vi "TDMS Playback Functional.vi"(1 "Scale Factor Linear":dbl=1.1934598400763813e-07, 4 "IQ Swap Enabled":bool=TRUE, 5 "IQ Rate (S/s)":dbl=25000000.0 format="%#_3p", 6 "pre filter gain":dbl, 7 "channel name (iq/qi)":string="qi", 8 "error in":errorcluster={"status"=FALSE, "code"=373504, "source"="niRFSG Close.vi<ERR>DSP overflow detected. The output waveform was clipped. Reduce the Arb Pre-filter Gain to eliminate overflow."}, 9 "Output Power (dBm)":dbl=10.0 format="%#_3p", 10 "Carrier (Hz)":dbl=3550000000.0 format="%#_3p", 11 "Path":path) -> (0 "error out":errorcluster={"status"=FALSE, "code"=373504, "source"="niRFSG Close.vi<ERR>DSP overflow detected. The output waveform was clipped. Reduce the Arb Pre-filter Gain to eliminate overflow."}, 2 "Playback Progress":i32(slide)=383 scale=-1.0..536.0)   [LabVIEW 2017]
uses:
  <instrlib>/niRFSG/niRFSG.llb/niRFSG Write Arb Waveform (Complex DBL).vi
  MainVI/GlobalVariableS.vi
  <vilib>/FPGAPlugInAG/Dynamic/niLvFpga_Close_Dynamic.vi
  <vilib>/rvi/interface/nirviCloseFPGA/nirviCloseFPGA.xnode
panel:
  out "result string 2":string
  out "20 log (scale Factor_Linear)":dbl=-138.46384380841334
  in  "RF:LO Out Enabled":bool
  in  "RF:External Gain (dB)":dbl
  in  "RF:Peak Power Adjustment (dB)":dbl
  out "samples":u32=769639589
  out "number of pending reads 1":u32=8
  out "empty elements":u32=134217728
  out "dma fullness":u32=48764
  out "number of pending reads 2":u32=1
  out "# of elements in host buffer avail for writing":u32=65536
  out "peak fullness":u32
  out "fullness":u32=65536
  out "Completion Loop":i32=3891
  out "fpga peak":u32(slide)=272 scale=-1.0..65536.0
  in  "Monitor Buffer Fullness":bool=TRUE
  out "file peak":u32(slide)=2 scale=0.0..8.0
  out "host peak":u32(slide)=1024 scale=-1.0..134217728.0
  out "File Read Buffer Fullness":u32(slide)=1 scale=0.0..8.0
  out "DMA Host Buffer Emptiness":u32(slide) scale=-1.0..134217728.0
  out "DMA FPGA Buffer Emptiness":u32(slide)=424 scale=-1.0..65536.0
  out "Underflow Detected":bool
  in  "stop button":bool
  in  "Read Block Size (MB)":u32=32 caption="Chunk Size (S)" format="%.0f MB"
  in  "chunks":u32=16 caption="DMA Host Buffer Depth (Blocks)" format="%.0p"
  in  "VST Resource":string="VST"
  # "RF Playback Configuration"
  # "VST Internal FPGA Status"
  # "File"
  # "Current"
  # "Peak"
  # "Current"
  # "Peak"
  # "RF"
  # "Current"
  # "Peak"
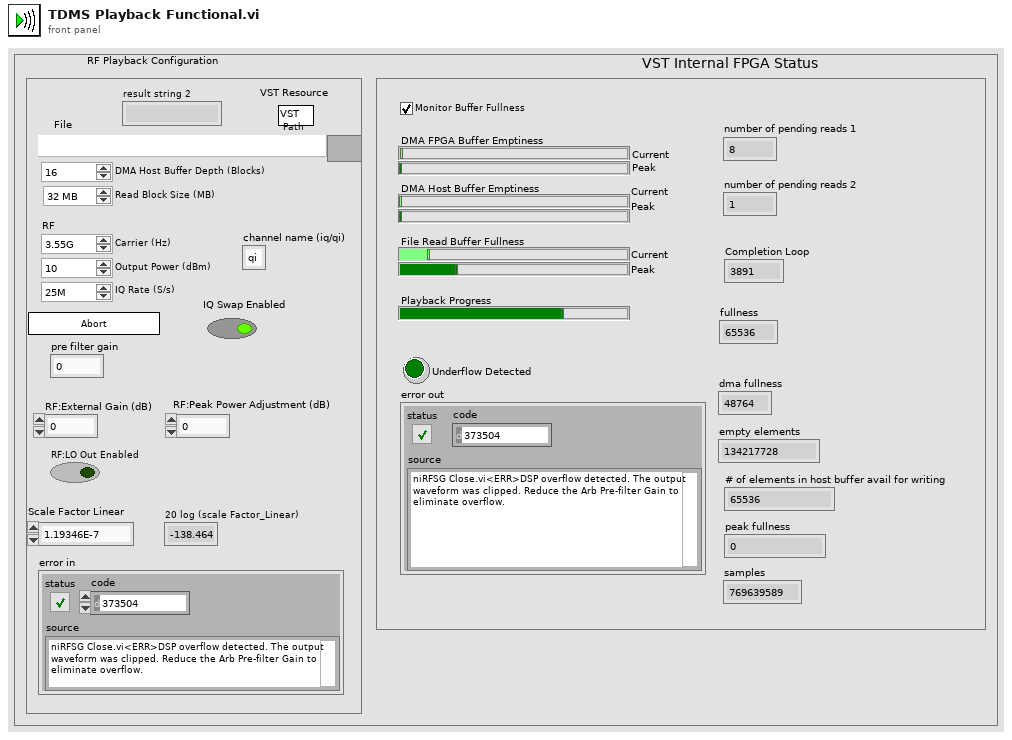
[diagram p1: front panel]
types:
  T1 = enum16{"open", "open or create", "create or replace", "create", "open (read-only)"}
  T2 = cluster{"underflow":bool, "underflows":u32, "samples":u32}
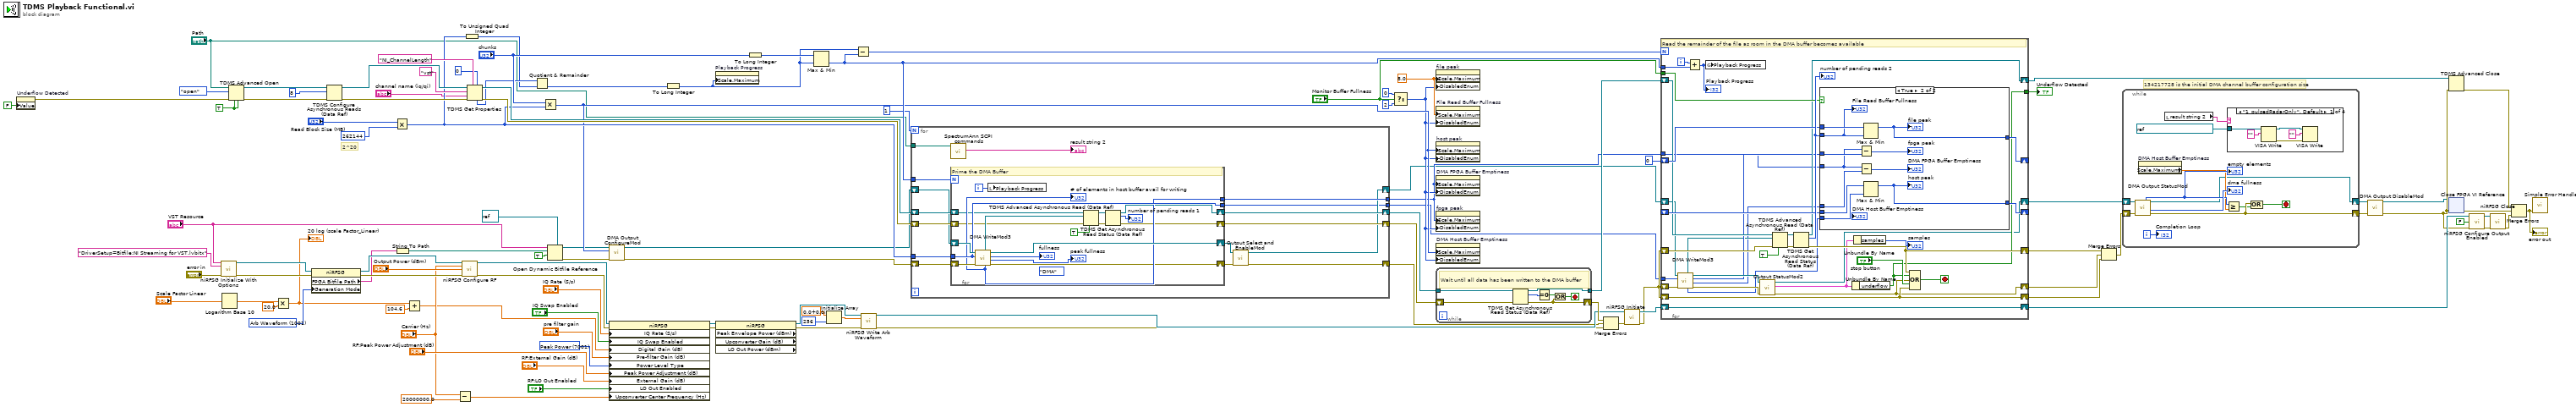
[diagram p0: block diagram]
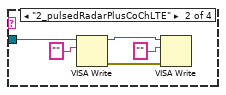
[diagram p3: hidden frame]
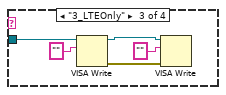
[diagram p4: hidden frame]
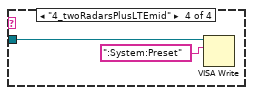
[diagram p5: hidden frame]
diagram:
  w24 = 7001 items=["Average Power"=7000, "Peak Power"=7001] ("RF:Power Level Type")
  w48 = 8.0 ("Scale.Range:Maximum")
  w14 = TRUE ("disable buffering? (T)")
  w102 = 1001 items=["CW"=1000, "Arb Waveform"=1001, "Script"=1002] ("Arb:Generation Mode")
  # "134217728 is the initial DMA channel buffer configuration size"
  # "2^20"
  n1 = property on="Underflow Detected" class="Bool (strict)"("Value"=FALSE ("Underflow Detected")) -> (error out=w46:errorcluster)  [unwired: 2 in, 1 out]
  n2 = call <instrlib>:"niRFSG Initialize With Options.vi"("resource name"="VST Resource", "option string"="DriverSetup=Bitfile:NI Streaming for VST.lvbitx", "error in"="error in") -> ("instrument handle"=w107:refnum<k15>, "error out"=w108:errorcluster)  [unwired: 11 in]
  n3 = Logarithm Base 10(1:"Scale Factor Linear") -> (0:w9:dbl)
  n4 = TDMS Advanced Open(4:w14, 6:w14, 8:w46, 10:T1."open" ("operation (0:open)"), 11:"Path") -> (0:w98:errorcluster, 3:w97:refnum<k34>)  [unwired: 1 out]
  n5 = Multiply(x=w9, y=20.0) -> (x*y=w8:dbl)
  "20 log (scale Factor_Linear)" <- w8
  n6 = property class="niRFSG"(reference=w107, error in=w108, "Generation Mode"=w102) -> (reference out=w105:refnum<k15>, error out=w106:errorcluster, "FPGA Bitfile Path"=w104:string)
  n7 = TDMS Configure Asynchronous Reads (Data Ref)(8:w98, 10:u32 8 ("max asynchronous reads (4)"), 11:w97) -> (0:w87:errorcluster, 3:w88:refnum<k34>)  [unwired: 2 in]
  n8 = Multiply(x="Read Block Size (MB)", y=u32 262144) -> (x*y=w56:u32)
  n9 = String To Path(string=w104) -> (path=w36:path)
  n10 = Add(x=w8, y=104.6) -> (x+y=w4:dbl)
  n11 = Subtract(x="Carrier (Hz)", y=20000000.0) -> (x-y=w10:dbl)
  n12 = call <instrlib>:"niRFSG Configure RF.vi"("instrument handle"=w105, "frequency (Hz)"="Carrier (Hz)", "power level (dBm)"="Output Power (dBm)", "error in"=w106) -> ("instrument handle out"=w23:refnum<k15>, "error out"=w22:errorcluster)  [unwired: 10 in]
  n13 = To Unsigned Quad Integer(1:w56) -> (0:w59:u64)
  n14 = TDMS Get Properties(5:u64 0, 7:"NI_ChannelLength" ("property name"), 8:w87, 9:"channel name (iq/qi)", 10:"vst" ("group name"), 11:w88) -> (0:w85:errorcluster, 3:w86:refnum<k34>, 4:w64:u64)  [unwired: 3 out]
  n15 = Quotient & Remainder(x=w64, y=w59) -> (floor(x/y)=w63:u64)  [unwired: 1 out]
  n16 = Multiply(x="chunks", y=w56) -> (x*y=w54:u32)
  n17 = Open Dynamic Bitfile Reference(0:"VST Resource", 1:w36, 2:TRUE ("Run When Loaded"), 4:refnum<k20> refnum ("Type")) -> (5:w27:refnum<k20>, 8:w26:errorcluster)  [unwired: 1 in]
  n18 = call "DMA Output ConfigureMod.vi"("error in (no error)"=w26, "depth"=w54, "Refnum in"=w27) -> ("error out"=w44:errorcluster, "Refnum out"=w43:refnum<k20>)  [unwired: 7 in]
  n19 = property class="niRFSG"(reference=w23, error in=w22, "IQ Rate (S/s)"="IQ Rate (S/s)", "IQ Swap Enabled"="IQ Swap Enabled", "Digital Gain (dB)"=w4, "Pre-filter Gain (dB)"="pre filter gain", "Power Level Type"=w24, "Peak Power Adjustment (dB)"="RF:Peak Power Adjustment (dB)", "External Gain (dB)"="RF:External Gain (dB)", "LO Out Enabled"="RF:LO Out Enabled", "Upconverter Center Frequency (Hz)"=w10) -> (reference out=w21:refnum<k15>, error out=w19:errorcluster)
  n20 = To Long Integer(number=w63) -> (32bit integer=w49:i32)
  n21 = property on="Playback Progress" class="Slide (strict)"("Scale.Maximum"=w49) -> ()  [unwired: 2 in, 2 out]
  n22 = property class="niRFSG" props=["Peak Envelope Power (dBm)", "Upconverter Gain (dB)", "LO Out Power (dBm)"](reference=w21, error in=w19) -> (reference out=w20:refnum<k15>, error out=w18:errorcluster)  [unwired: 3 out]
  n23 = To Long Integer(number="chunks") -> (32bit integer=w81:i32)
  n24 = Max & Min(x=w81, y=w49) -> (min(x,y)=w58:i32)  [unwired: 1 out]
  n25 = Initialize Array(cdb 0.0+0.0i ("element"), 256 ("dimension size")) -> (w32:cdb[])
  n26 = Subtract(x=w49, y=w58) -> (x-y=w57:i32)
  n27 = call-poly <instrlib>:"niRFSG Write Arb Waveform.vi"("instrument handle"=w20, "waveform data"=w32, "error in"=w18) -> ("instrument handle out"=w79:refnum<k15>, "error out"=w78:errorcluster)  [unwired: 11 in]
  n28 = for {
    N: 1 -> [_]
    tunnel: w58 -> [w121]
    tunnel: w56 -> [w120]
    tunnel: [w116] -> w41
    tunnel: [w114] -> w35
    shift-right: [w125] -> w96
    shift-left: w86 -> [w123]
    shift-right: [w124] -> w95
    shift-left: w85 -> [w122]
    shift-right: [w119] -> w45
    shift-left: w44 -> [w118]
    shift-right: [w115] -> w38
    shift-left: w43 -> [w117]
    tunnel: "Path" -> [w110]
    n29 = call "SpectrumAnn SCPI commands.vi"("Path"=w110) -> ("result string"=→"result string 2":string)  [unwired: 8 in, 2 out]
    n30 = for {
      N: w121 -> [_]
      shift-right: [w130] -> w124
      shift-left: w122 -> [w126]
      shift-right: [w133] -> w113
      shift-left: w118 -> [w142]
      shift-right: [w129] -> w125
      shift-left: w123 -> [w127]
      shift-right: [w141] -> w112
      shift-left: w117 -> [w143]
      tunnel: w120 -> [w140]
      tunnel: [w140] -> w114
      tunnel: [w138] -> w116
      i -> [w139]
      (unwired) enum16{"none", "DMA", "local", "P2P", "DIO"}."DMA" ("stream select")
      # "Prime the DMA Buffer"
      n31 = call "DMA WriteMod3.vi"("error in (no error)"=w142, "number of elements"=w140, "Refnum in"=w143) -> ("error out"=w133:errorcluster, "peak fullness"=→"peak fullness":u32, "fullness"=→"fullness":u32, "Refnum out"=w141:refnum<k20>, "empty elements remaining"=w138:u32, "Write Region Reference"=w137:refnum<data-value>)  [unwired: 3 in]
      "# of elements in host buffer avail for writing" <- w138
      n32 = local write "Playback Progress"(w139) -> ()
      n33 = TDMS Advanced Asynchronous Read (Data Ref)(6:TRUE ("auto delete reference? (T)"), 8:w126, 10:w137, 11:w127) -> (0:w131:errorcluster, 3:w132:refnum<k34>)  [unwired: 1 out]
      n34 = TDMS Get Asynchronous Read Status (Data Ref)(8:w131, 11:w132) -> (0:w130:errorcluster, 2:→"number of pending reads 1":u32, 3:w129:refnum<k34>)
    }
    n35 = call "Output Select and EnableMod.vi"("error in (no error)"=w113, "Refnum in"=w112) -> ("error out"=w119:errorcluster, "Refnum out"=w115:refnum<k20>)  [unwired: 8 in]
  }
  n36 = Select(t=0, s="Monitor Buffer Fullness", f=2) -> (s? t:f=w42:i32)
  n37 = property on="file peak" class="Slide (strict)"("Scale.Maximum"=w48, "DisabledEnum"=w42) -> ()  [unwired: 2 in, 2 out]
  n38 = property on="File Read Buffer Fullness" class="Slide (strict)"("Scale.Maximum"=w48, "DisabledEnum"=w42) -> ()  [unwired: 2 in, 2 out]
  n39 = property on="host peak" class="Slide (strict)"("Scale.Maximum"=w54, "DisabledEnum"=w42) -> ()  [unwired: 2 in, 2 out]
  n40 = property on="DMA FPGA Buffer Emptiness" class="Slide (strict)"("Scale.Maximum"=w41, "DisabledEnum"=w42) -> ()  [unwired: 2 in, 2 out]
  n41 = property on="fpga peak" class="Slide (strict)"("Scale.Maximum"=w41, "DisabledEnum"=w42) -> ()  [unwired: 2 in, 2 out]
  n42 = property on="DMA Host Buffer Emptiness" class="Slide (strict)"("Scale.Maximum"=w54, "DisabledEnum"=w42) -> ()  [unwired: 2 in, 2 out]
  n43 = while {
    tunnel: w96 -> [w149]
    shift-right: [w145] -> w92
    shift-left: w95 -> [w150]
    tunnel: [w147] -> w91
    stop <- w146 stop-if-true
    # "Wait until all data has been written to the DMA buffer"
    n44 = TDMS Get Asynchronous Read Status (Data Ref)(8:w150, 11:w149) -> (0:w145:errorcluster, 2:w148:u32, 3:w147:refnum<k34>)
    n45 = Equal To 0?(x=w148) -> (x = 0?=w144:bool)
    n46 = Or(x=w144, y=w145) -> (x .or. y?=w146:bool)
  }
  n47 = Merge Errors(w92, w45, w78) -> (w94:errorcluster)
  n48 = call <instrlib>:"niRFSG Initiate.vi"("instrument handle"=w79, "error in"=w94) -> ("instrument handle out"=w93:refnum<k15>, "error out"=w80:errorcluster)  [unwired: 12 in]
  n49 = for {
    N: w57 -> [_]
    shift-right: [w184] -> w67
    shift-left: w80 -> [w184]
    shift-right: [w165] -> w68
    shift-left: w80 -> [w172]
    shift-right: [w168] -> w69
    shift-left: w80 -> [w173]
    shift-right: [w164] -> w89
    shift-left: w91 -> [w171]
    shift-right: [w185] -> w75
    shift-left: w93 -> [w185]
    tunnel: w58 -> [w181]
    tunnel: w35 -> [w158]
    tunnel: [w162] -> w55
    shift-right: [w178] -> _
    shift-left: u32 0 -> [w177]
    shift-right: [w176] -> _
    shift-left: _ -> [w175]
    tunnel: "Monitor Buffer Fullness" -> [w174]
    tunnel: w41 -> [w161]
    shift-right: [w157] -> w37
    shift-left: w38 -> [w159]
    i -> [w180]
    stop <- w182 stop-if-true
    # "Read the remainder of the file as room in the DMA buffer becomes available"
    n50 = call "DMA WriteMod3.vi"("error in (no error)"=w173, "number of elements"=w158, "Refnum in"=w159) -> ("error out"=w169:errorcluster, "peak fullness"=w154:u32, "fullness"=w163:u32, "Refnum out"=w170:refnum<k20>, "empty elements remaining"=w156:u32, "Write Region Reference"=w155:refnum<data-value>)  [unwired: 3 in]
    n51 = Add(x=w180, y=w181) -> (x+y=w151:i32)
    "Playback Progress" <- w151
    n52 = global write "GlobalVariableS.vi" "Playback Progress"(w151) -> ()
    n53 = call "Output StatusMod2.vi"("error in (no error)"=w169, "Refnum in"=w170) -> ("error out"=w168:errorcluster, "status"=w153:T2, "Refnum out"=w157:refnum<k20>)  [unwired: 7 in]
    n54 = TDMS Advanced Asynchronous Read (Data Ref)(6:TRUE ("auto delete reference? (T)"), 8:w172, 10:w155, 11:w171) -> (0:w167:errorcluster, 3:w166:refnum<k34>)  [unwired: 1 out]
    n55 = TDMS Get Asynchronous Read Status (Data Ref)(8:w167, 11:w166) -> (0:w165:errorcluster, 2:w179:u32, 3:w164:refnum<k34>)
    "number of pending reads 2" <- w179
    n56 = case shown="True" w174 {
      tunnel: w179 -> [_ w195]
      tunnel: [_ w193] -> w178
      tunnel: w177 -> [_ w196]
      tunnel: [_ w192] -> w176
      tunnel: w175 -> [_ w194]
      tunnel: w154 -> [_ w188]
      tunnel: w163 -> [_ w190]
      tunnel: w156 -> [_ w191]
      tunnel: w161 -> [_ w187]
      frame False {
      }
      frame True {
        n57 = Subtract(x=w187, y=w190) -> (x-y=→"fpga peak":u32)
        n58 = Subtract(x=w187, y=w188) -> (x-y=→"DMA FPGA Buffer Emptiness":u32)
        n59 = Max & Min(x=w196, y=w195) -> (max(x,y)=w193:u32)  [unwired: 1 out]
        "file peak" <- w193
        n60 = Max & Min(x=w194, y=w191) -> (max(x,y)=w192:u32)  [unwired: 1 out]
        "host peak" <- w192
        "File Read Buffer Fullness" <- w195
      }
    }
    n61 = Unbundle By Name(w153) -> ("underflow"=w162:bool)
    n62 = Unbundle By Name(w153) -> ("samples"=→"samples":u32)
    n63 = Compound Arithmetic op=OR(w165, w162, w168, "stop button", w184) -> (w182:bool)
  }
  "Underflow Detected" <- w55
  n64 = Merge Errors(w68, w69, w67) -> (w90:errorcluster)
  n65 = while {
    shift-right: [w204] -> w77
    shift-left: w90 -> [w208]
    shift-right: [w199] -> w76
    shift-left: w37 -> [w207]
    i -> [w206]
    stop <- w205 stop-if-true
    n66 = call "DMA Output StatusMod.vi"("error in (no error)"=w208, "Refnum in"=w207) -> ("error out"=w204:errorcluster, "dma fullness"=→"dma fullness":u32, "Refnum out"=w199:refnum<k20>, "empty elements"=w201:u32)  [unwired: 5 in, 1 out]
    "empty elements" <- w201
    n67 = property on="DMA Host Buffer Emptiness" class="Slide (strict)"() -> ("Scale.Maximum"=w200:dbl)  [unwired: 2 in, 2 out]
    n68 = local read "result string 2"() -> (w197:string)
    n69 = Greater Or Equal?(x=w201, y=w200) -> (x >= y?=w203:bool)
    n70 = case shown="\"1_pulsedRadarOnly\", Default" w197 {
      tunnel: refnum<visa-resource-name> "SpecAnn-9010A-20100" ("VISA resource name") -> [w209 w214 w219 w225]
      frame "1_pulsedRadarOnly", Default {
        n71 = VISA Write(VISA resource name=w209, write buffer="") -> (VISA resource name out=w212:refnum<visa-resource-name>, error out=w211:errorcluster)  [unwired: 1 in, 1 out]
        n72 = VISA Write(VISA resource name=w212, write buffer="", error in (no error)=w211) -> ()  [unwired: 3 out]
      }
      frame "2_pulsedRadarPlusCoChLTE" {
        n73 = VISA Write(VISA resource name=w214, write buffer="") -> (VISA resource name out=w217:refnum<visa-resource-name>, error out=w216:errorcluster)  [unwired: 1 in, 1 out]
        n74 = VISA Write(VISA resource name=w217, write buffer="", error in (no error)=w216) -> ()  [unwired: 3 out]
      }
      frame "3_LTEOnly" {
        n75 = VISA Write(VISA resource name=w219, write buffer="") -> (VISA resource name out=w222:refnum<visa-resource-name>, error out=w221:errorcluster)  [unwired: 1 in, 1 out]
        n76 = VISA Write(VISA resource name=w222, write buffer="", error in (no error)=w221) -> ()  [unwired: 3 out]
      }
      frame "4_twoRadarsPlusLTEmid" {
        n77 = VISA Write(VISA resource name=w225, write buffer=":System:Preset") -> ()  [unwired: 1 in, 3 out]
      }
    }
    n78 = Compound Arithmetic op=OR(w204, w203) -> (w205:bool)
    "Completion Loop" <- w206
  }
  n79 = call "DMA Output DisableMod.vi"("error in (no error)"=w77, "Refnum in"=w76) -> ("error out"=w29:errorcluster, "Refnum out"=w28:refnum<k20>)  [unwired: 8 in]
  n80 = TDMS Advanced Close(8:w29, 11:w89) -> (0:w62:errorcluster)  [unwired: 2 in, 1 out]
  n81 = xnode "Close FPGA VI Reference"("FPGA VI Reference In"=w28, "error in"=w29) -> ("error out"=w61:errorcluster)
  n82 = call <instrlib>:"niRFSG Configure Output Enabled.vi"("instrument handle"=w75, "output enabled"=FALSE, "error in"=w29) -> ("instrument handle out"=w73:refnum<k15>, "error out"=w74:errorcluster)  [unwired: 11 in]
  n83 = call <instrlib>:"niRFSG Close.vi"("instrument handle"=w73, "error in"=w74) -> ("error out"=w60:errorcluster)  [unwired: 13 in]
  n84 = Merge Errors(w62, w61, w60) -> (w30:errorcluster)
  "error out" <- w30
  n85 = call <vilib>:"Simple Error Handler.vi"("error in (no error)"=w30) -> ()  [unwired: 4 in, 5 out]
